vi "executesql.vi"(7 "Return Data (T)":bool=TRUE, 8 "Command Text":string) -> (3 "error out":errorcluster, 5 "Data":string[][](array[string]))   [LabVIEW 2014]
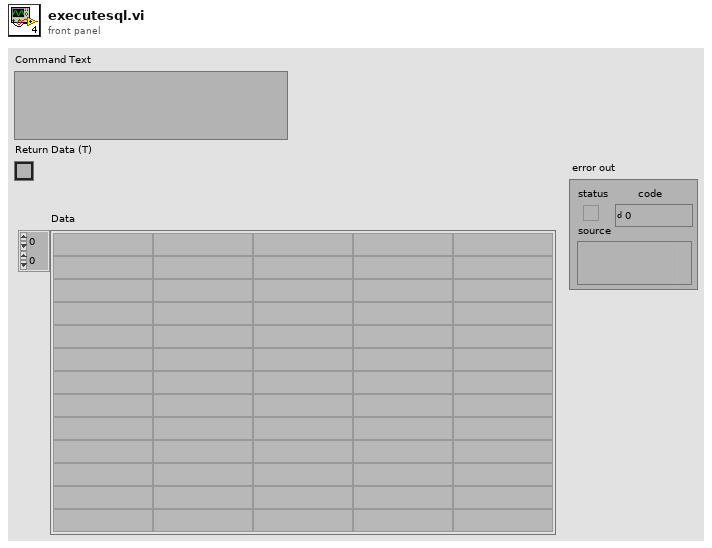
[diagram p1: front panel]
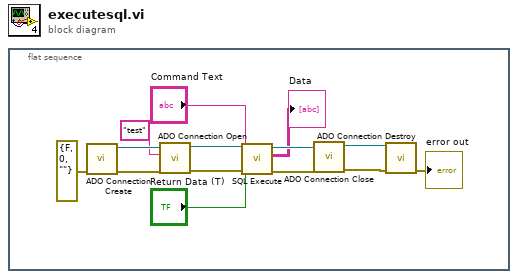
[diagram p0: block diagram]
diagram:
  n1 = flat-sequence {
    frame #0 {
      n2 = call <userlib>:"ADO Connection Create.vi"("error in (no error)"=errorcluster {"status"=FALSE, "code"=0, "source"=""}) -> ("error out"=w13:errorcluster, "ADODB._Connection Out"=w14:refnum<k7>)  [unwired: 9 in]
      n3 = call <userlib>:"ADO Connection Open.vi"("error in (no error)"=w13, "ConnectionString"="test", "ADODB._Connection In"=w14) -> ("error out"=w9:errorcluster, "ADODB._Connection Out"=w10:refnum<k7>)  [unwired: 7 in]
      n4 = call <userlib>:"SQL Execute.vi"("error in (no error)"=w9, "Return Data (T)"="Return Data (T)", "Command Text"="Command Text", "ADODB._Connection In"=w10) -> ("error out"=w6:errorcluster, "Data"=→"Data":string[][], "ADODB._Connection Out"=w8:refnum<k7>)  [unwired: 4 in, 1 out]
      n5 = call <userlib>:"ADO Connection Close.vi"("error in (no error)"=w6, "ADODB._Connection In"=w8) -> ("error out"=w5:errorcluster, "ADODB._Connection Out"=w7:refnum<k7>)  [unwired: 8 in]
      n6 = call <userlib>:"ADO Connection Destroy.vi"("error in (no error)"=w5, "ADODB._Connection In"=w7) -> ("error out"=→"error out":errorcluster)  [unwired: 9 in]
    }
  }
